vi "Is Created Queue.vi"(10 "Created Queue Alias":string, 11 "Queue jettl in":refnum<class "Queue jettl.lvclass">) -> (2 "Is Created Queue?":bool, 3 "Queue jettl out":refnum<class "Queue jettl.lvclass">)   [LabVIEW 2021, in "jettl.lvlib" / "Queue jettl.lvclass"]
uses:
  Queue jettl.lvclass
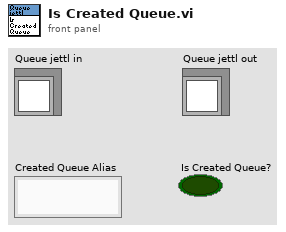
[diagram p1: front panel]
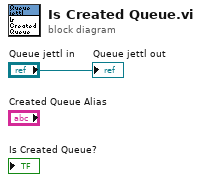
[diagram p0: block diagram]
diagram:
  "Queue jettl out" <- "Queue jettl in"
